vi "Verify Pwd.vi"(1 "Encrypted Password":string, 2 "Password Input":string) -> (0 "Valid":bool)   [LabVIEW 2016, in "UserPwd DB.lvlib" / "UserPwd DB.lvclass"]
uses:
  <userlib>/Common Components/UserPwd DB/UserPwd DB/UserPwd DB.lvclass
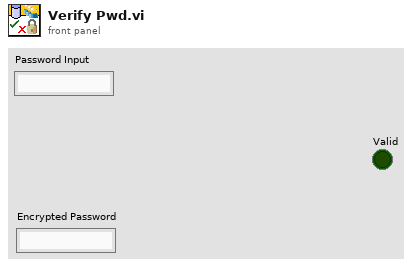
[diagram p1: front panel]
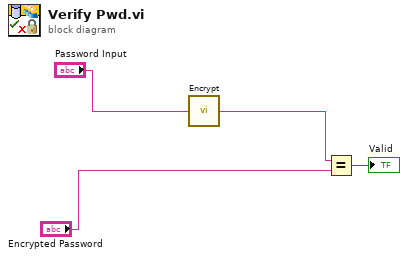
[diagram p0: block diagram]
diagram:
  n1 = call <userlib>:"Encrypt.vi"("String"="Password Input") -> ("Encrypted String"=w3:string)
  n2 = Equal?(x=w3, y="Encrypted Password") -> (x = y?=→"Valid":bool)
